vi "Test_Interpolate_ArrayTable.vi"() -> ()   [LabVIEW 2019]
uses:
  <vilib>/Analysis/6fits.llb/Curve Fitting Criteria.ctl
  <vilib>/Analysis/6fits.llb/General Linear Fit Algorithm.ctl
  <vilib>/Analysis/NI_AALPro.lvlib
panel:
  in  "algorithm":T1 items=["SVD", "Givens", "Givens2", "Householder", "LU Decomposition", "Cholesky", "SVD for Rank Deficient H"]
  in  "method":T2 items=["Least Square", "Least Absolute Residual", "Bisquare"]
  out "Polynomial Coefficients":dbl[](array[numeric])
  out "Best Polynomial Fit":dbl[](array[numeric])
  in  "array":dbl[][](array[numeric])=[[45.0, 5800.0], [51.0, 5300.0], [70.0, 4900.0], [80.0, 4850.0], [130.0, 4750.0], [150.0, 4675.0], [180.0, 4650.0]]
  out "Test Plot":cluster{dbl[], dbl[]}[](graph)
  in  "StopValue":dbl=250.0
  in  "StartValue":dbl
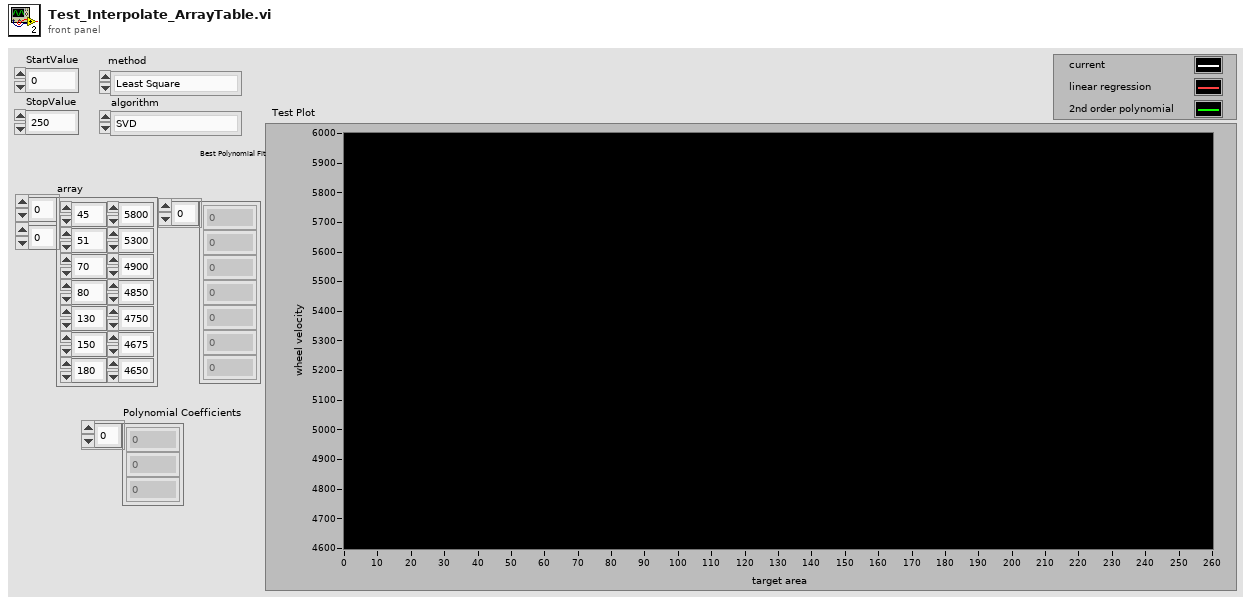
[diagram p1: front panel]
types:
  T1 = typedef "NI_AALPro.lvlib/General Linear Fit Algorithm.ctl" = u16
  T2 = typedef "NI_AALPro.lvlib/Curve Fitting Criteria.ctl" = u16
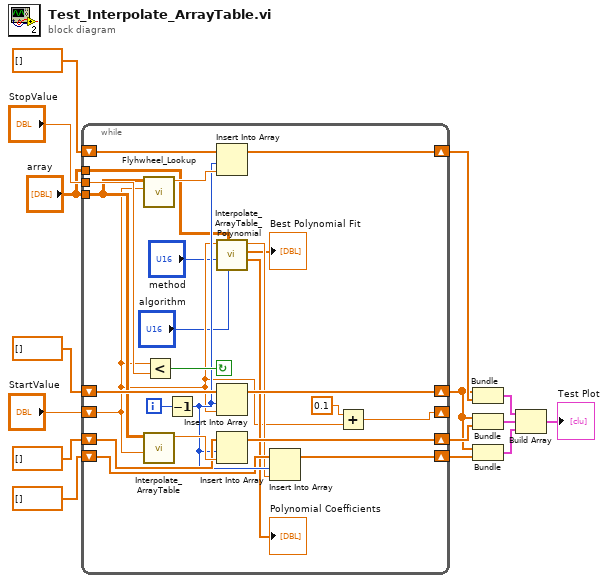
[diagram p0: block diagram]
diagram:
  n1 = while {
    shift-right: [w38] -> _
    shift-left: "StartValue" -> [w19]
    tunnel: "StopValue" -> [w37]
    shift-right: [w32] -> w4
    shift-left: dbl[] [] -> [w34]
    shift-right: [w31] -> w6
    shift-left: dbl[] [] -> [w33]
    shift-right: [w28] -> w7
    shift-left: dbl[] [] -> [w29]
    tunnel: "array" -> [w26]
    shift-right: [w23] -> w3
    shift-left: dbl[] [] -> [w24]
    tunnel: "array" -> [w16]
    i -> [w35]
    stop <- w36 continue-if-true
    n2 = call "Flyhwheel_Lookup.vi"("search_value"=w19, "array"=w26) -> ("RPM output"=w27:dbl)  [unwired: 9 in]
    n3 = call "Interpolate_ArrayTable.vi"("Desired_Distance"=w19, "array"=w26) -> ("RPM"=w30:dbl)  [unwired: 9 in]
    n4 = Less?(x=w19, y=w37) -> (x < y?=w36:bool)
    n5 = Decrement(x=w35) -> (x-1=w25:i32)
    n6 = Insert Into Array(array=w33, index=w25, new element=w27) -> (w31:dbl[])
    n7 = call "Interpolate_ArrayTable_Polynomial.vi"("algorithm"="algorithm", "array"=w16, "method"="method", "Desired_Distance"=w19) -> ("Polynomial Coefficients"=→"Polynomial Coefficients":dbl[], "Best Polynomial Fit"=→"Best Polynomial Fit":dbl[], "RPM"=w22:dbl)  [unwired: 5 in]
    n8 = Insert Into Array(array=w34, index=w25, new element=w19) -> (w32:dbl[])
    n9 = Insert Into Array(array=w29, index=w25, new element=w30) -> (w28:dbl[])
    n10 = Insert Into Array(array=w24, index=w25, new element=w22) -> (w23:dbl[])
    n11 = Add(x=0.1, y=w19) -> (x+y=w38:dbl)
  }
  n12 = Bundle(w4, w6) -> (w9:cluster{dbl[], dbl[]})  [unwired: 1 in]
  n13 = Bundle(w4, w7) -> (w10:cluster{dbl[], dbl[]})  [unwired: 1 in]
  n14 = Bundle(w4, w3) -> (w2:cluster{dbl[], dbl[]})  [unwired: 1 in]
  n15 = Build Array(w9, w10, w2) -> (→"Test Plot":cluster{dbl[], dbl[]}[])
